vi "TetrixMorotControl_Main.vi"() -> ()   [LabVIEW 2014]
panel:
  in  "Motor 1 Power (-100 to 100)\n0 = Stop/Brake\n-128 = Stop/Coast":i8(slide) scale=-100.0..100.0
  in  "Motor 2 Power (-100 to 100)\n0 = Stop/Brake\n-128 = Stop/Coast":i8(slide) scale=-100.0..100.0
  in  "Controller Daisy Chain Position: 1 - 5":u8=1
  in  "Power (-100 to 100)\n0 = Stop/Brake\n-128 = Stop/Coast":i8(slide) scale=-100.0..100.0
  in  "Encoder Target: 360 = 1 motor shaft revolution":i32
  in  "Controller Daisy Chain Position: 1 - 4":u8=2 min=1 max=4
  in  "Select Channel":string(combo)="Motor 1"
  in  "정지":bool
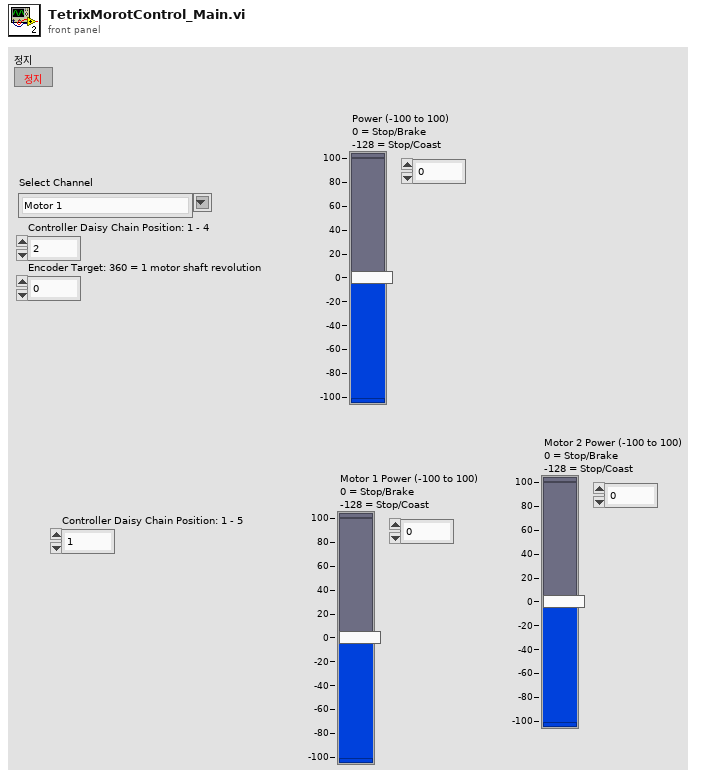
[diagram p1: front panel]
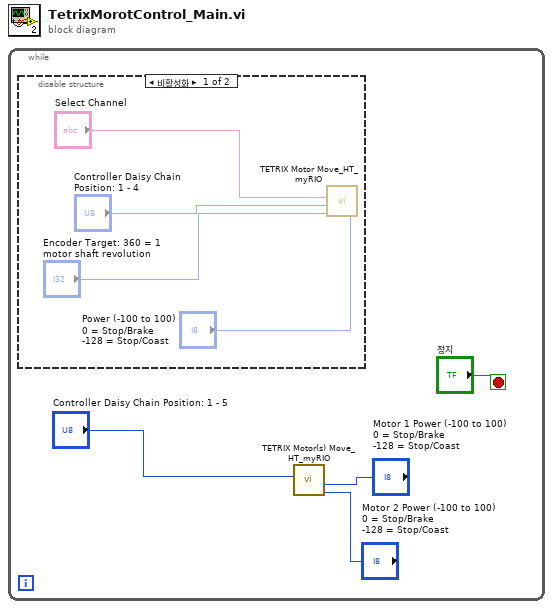
[diagram p0: block diagram]
diagram:
  n1 = while {
    stop <- "정지" stop-if-true
    n2 = disable-structure shown="비활성화" {
      frame Disabled {
        n3 = call <vilib>:"TETRIX Motor Move_HT_myRIO.vi"("Power (-100 to 100)\n0 = Stop/Brake\n-128 = Stop/Coast"="Power (-100 to 100)\n0 = Stop/Brake\n-128 = Stop/Coast", "Encoder Target: 360 = 1 motor shaft revolution"="Encoder Target: 360 = 1 motor shaft revolution", "Controller Daisy Chain Position: 1 - 4"="Controller Daisy Chain Position: 1 - 4", "Select Channel"="Select Channel") -> ()  [unwired: 3 in, 1 out]
      }
      frame Enabled {
      }
    }
    n4 = call <vilib>:"TETRIX Motor(s) Move_HT_myRIO.vi"("Motor 2 Power (-100 to 100)\n0 = Stop/Brake\n-128 = Stop/Coast"="Motor 2 Power (-100 to 100)\n0 = Stop/Brake\n-128 = Stop/Coast", "Motor 1 Power (-100 to 100)\n0 = Stop/Brake\n-128 = Stop/Coast"="Motor 1 Power (-100 to 100)\n0 = Stop/Brake\n-128 = Stop/Coast", "Controller Daisy Chain Position: 1 - 4"="Controller Daisy Chain Position: 1 - 5") -> ()  [unwired: 6 in, 1 out]
  }
